vi "DAQ - READ- Multiple waveforms from multiple channels.vi"(4 "Digital Pause Trigger Pause When":i32(ring)=10192 caption="Pause When" items=["High"=10192, "Low"=10214], 6 "Digital Trigger Source":tag="/Dev1/PFI0" caption="Trigger Source", 8 "error in":errorcluster, 10 "Sample Rate":dbl=1000.0, 11 "Task/channels in":refnum<k21>) -> (0 "error out":errorcluster, 2 "data":waveform(dbl)[](array[waveform]), 3 "task out":refnum<k21>)   [LabVIEW 2017]
uses:
  <vilib>/Utility/error.llb/DialogType.ctl
  <vilib>/DAQmx/read.llb/DAQmx Read (Analog 1D Wfm NChan NSamp).vi
  <vilib>/DAQmx/configure/timing.llb/DAQmx Timing (Sample Clock).vi
  <vilib>/DAQmx/configure/trigger.llb/DAQmx Start Trigger (Digital Edge).vi
  <vilib>/DAQmx/miscellaneous.llb/DAQmx Fill In Error Info.vi
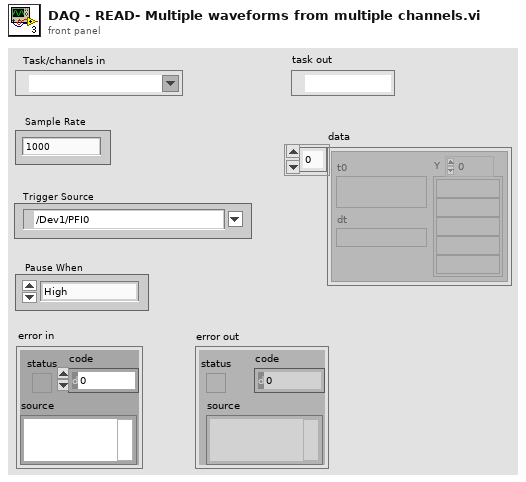
[diagram p1: front panel]
types:
  T1 = typedef "DialogType.ctl" = u16
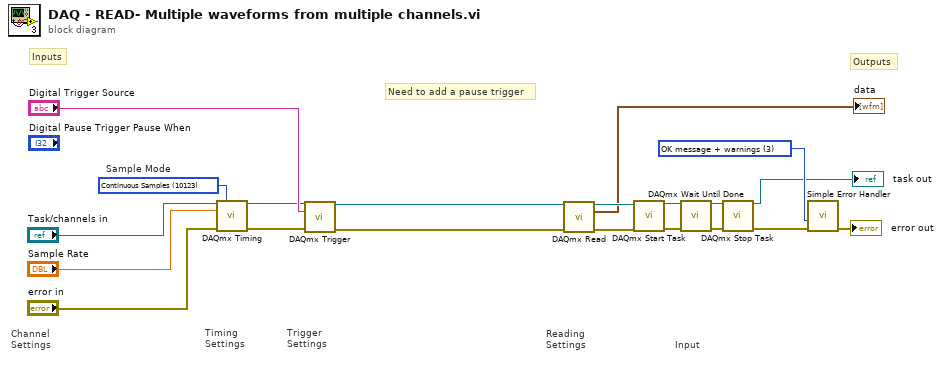
[diagram p0: block diagram]
diagram:
  w11 = T1 3 items=["no dialog", "OK message", "continue or stop message", "OK message + warnings", "continue/stop + warnings"] ("type of dialog (OK msg:1)")
  w18 = 10123 items=["Finite Samples"=10178, "Continuous Samples"=10123, "Hardware Timed Single Point"=12522]  # Sample Mode
  # "Need to add a pause trigger"
  # "Outputs"
  # "Inputs"
  # "Trigger \nSettings"
  # "Input"
  # "Reading\nSettings"
  # "Timing \nSettings"
  # "Channel \nSettings"
  n1 = call-poly <vilib>:"DAQmx Timing.vi"("task/channels in"="Task/channels in", "sample mode"=w18, "rate"="Sample Rate", "error in"="error in") -> ("task out"=w19:refnum<k21>, "error out"=w10:errorcluster)  [unwired: 10 in]
  n2 = call-poly <vilib>:"DAQmx Trigger.vi"("task/channels in"=w19, "source"="Digital Trigger Source", "error in"=w10) -> ("task out"=w2:refnum<k21>, "error out"=w1:errorcluster)  [unwired: 11 in]
  n3 = call-poly <vilib>:"DAQmx Read.vi"("task/channels in"=w2, "error in"=w1) -> ("task out"=w17:refnum<k21>, "data"=→"data":waveform(dbl)[], "error out"=w16:errorcluster)  [unwired: 11 in]
  n4 = call <vilib>:"DAQmx Start Task.vi"("task/channels in"=w17, "error in"=w16) -> ("task out"=w15:refnum<k21>, "error out"=w14:errorcluster)  [unwired: 12 in]
  n5 = call <vilib>:"DAQmx Wait Until Done.vi"("task/channels in"=w15, "error in"=w14) -> ("task out"=w13:refnum<k21>, "error out"=w12:errorcluster)  [unwired: 12 in]
  n6 = call <vilib>:"DAQmx Stop Task.vi"("task/channels in"=w13, "error in"=w12) -> ("task out"=→"task out":refnum<k21>, "error out"=w5:errorcluster)  [unwired: 12 in]
  n7 = call <vilib>:"Simple Error Handler.vi"("type of dialog (OK msg:1)"=w11, "error in (no error)"=w5) -> ("error out"=→"error out":errorcluster)  [unwired: 3 in, 4 out]
